vi "CreatePrivateEvents.vi"(8 "error in (no error)":errorcluster, 11 "LockinDAQ":refnum<class "Lockin.DAQ.lvclass">=refnum) -> (0 "error out":errorcluster, 3 "LockinDAQ out":refnum<class "Lockin.DAQ.lvclass">)   [LabVIEW 2016, in "Lockin.DAQ.lvclass"]
doc: "---------------------------------------------------------------\nJKI State Machine Objects™\nhttp://jki.net/state-machine-objects/\nCopyright (C) 2005-2015, JKI <info@jki.net>\nALL RIGHTS RESERVEDJKI State Machine Objects (SMO) 1.0.0.4\nJKI - JKI\nCopyright (c) 2015, JKI"
uses:
  Lockin.DAQ.lvclass
  Typedefs/PrivateEvents--Lockin.DAQ.setAOconfig.ctl
  Typedefs/AO.config-array.ctl
  Typedefs/AO.config-cluster.ctl
  Typedefs/446xAO-enum.ctl
  Typedefs/DAQType-enum.ctl
  Typedefs/PrivateEvents--Lockin.DAQ.setAIconfig.ctl
  Typedefs/AI.config-array.ctl
  Typedefs/AI.config-cluster.ctl
  Typedefs/AI.coupling-enum.ctl
  Typedefs/446xAI-enum.ctl
  Typedefs/AI Simulation-enum.ctl
  Typedefs/PrivateEvents--Lockin.DAQ.setAO.ctl
  Typedefs/AO-cluster.ctl
  Typedefs/Function-enum.ctl
  Typedefs/PrivateEvents--Lockin.DAQ.setREF.ctl
  Typedefs/REF-cluster.ctl
  Typedefs/PrivateEvents--Lockin.DAQ.setSampling.ctl
  Typedefs/Sampling.ctl
  Typedefs/Sample Mode--Ring.ctl
  Typedefs/PrivateEvents--Lockin.DAQ.setState.ctl
  Typedefs/Set State-enum.ctl
  Typedefs/PrivateEvents--Lockin.DAQ.setGain.ctl
  Typedefs/PrivateEvents--Lockin.DAQ.setSweep.ctl
  Typedefs/Sweep Configuration--Cluster.ctl
  Typedefs/Sweep Pattern--Enum.ctl
  Typedefs/PrivateEvents--Lockin.DAQ.measureOffset.ctl
  Typedefs/PrivateEvents--Lockin.DAQ.zeroOffset.ctl
  Typedefs/PrivateEvents--Lockin.DAQ.setPreFilter.ctl
  Typedefs/AI Prefilter-cluster.ctl
  Typedefs/PrivateEvents--Lockin.DAQ.autoContigureDAQ.ctl
  Typedefs/PrivateEvents--LockinDAQ.setCalibration.ctl
  Lockin.DAQ.lvclass/Lockin.DAQ.ctl
  Typedefs/PrivateEvents--LockinDAQ.Calibrate.ctl
  <vilib>/JKI/JKI SMO/SMO/SMO.lvclass
panel:
  # "For instructions on how to use the JKI State Machine Objects, examples and video tutorials, visit:\nhttp://jki.net/state-machine-objects/\n\nJKI State Machine Objects™\nhttp://jki.net/state-machine-objects/\nCopyright (C) 2005-2015, JKI <info@jki.net>\nALL RIGHTS RESERVED"
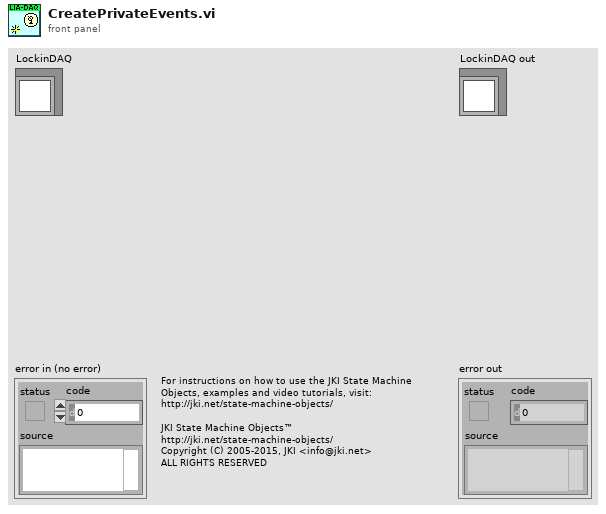
[diagram p1: front panel]
types:
  T1 = typedef "Lockin.DAQ.lvclass/PrivateEvents--LockinDAQ.setCalibration.ctl" = bool
  T2 = typedef "PrivateEvents--LockinDAQ.Calibrate.ctl" = bool
  T3 = typedef "Lockin.DAQ.lvclass/PrivateEvents--Lockin.DAQ.autoContigureDAQ.ctl" = bool
  T4 = typedef "Lockin.DAQ.lvclass/PrivateEvents--Lockin.DAQ.setPreFilter.ctl" = cluster{"PreFilter":T5}
  T5 = typedef "Lockin.DAQ.lvclass/AI Prefilter-cluster.ctl" = cluster{"60 Hz prefilter":bool, "LP prefilter":bool, "LP cutoff (Hz)":dbl}
  T6 = typedef "Lockin.DAQ.lvclass/PrivateEvents--Lockin.DAQ.zeroOffset.ctl" = bool
  T7 = typedef "Lockin.DAQ.lvclass/PrivateEvents--Lockin.DAQ.measureOffset.ctl" = bool
  T8 = typedef "Lockin.DAQ.lvclass/PrivateEvents--Lockin.DAQ.setSweep.ctl" = cluster{"setSweep":T9}
  T9 = typedef "Lockin.DAQ.lvclass/Sweep Configuration--Cluster.ctl" = cluster{"Sweep Lockin Time (s)":dbl, "Sweep IV Step (V)":dbl, "Initial Wait Time (s)":dbl, "Sweep Channel":i32[], "Sweep Start (V)":dbl[], "Sweep End (V)":dbl[], "Pattern":T10[], "Return to Start":bool}
  T10 = typedef "Lockin.DAQ.lvclass/Sweep Pattern--Enum.ctl" = enum16{"Ramp", "Ramp (RTS)", "Smooth Ramp", "Smooth Ramp (RTS)", "Frequency"}
  T11 = typedef "Lockin.DAQ.lvclass/PrivateEvents--Lockin.DAQ.setGain.ctl" = dbl[]
  T12 = typedef "Lockin.DAQ.lvclass/PrivateEvents--Lockin.DAQ.setState.ctl" = cluster{"setState":T13}
  T13 = typedef "Lockin.DAQ.lvclass/Set State-enum.ctl" = enum16{"start", "stop", "reset", "start sweep", "stop sweep"}
  T14 = typedef "Lockin.DAQ.lvclass/PrivateEvents--Lockin.DAQ.setSampling.ctl" = cluster{"Sampling":T15, "Sample Mode":T16, "AI Buffer Size (S)":i32, "Decimation":i32}
  T15 = typedef "Lockin.DAQ.lvclass/Sampling.ctl" = cluster{"Fs":dbl, "#s":i32}
  T16 = typedef "Lockin.DAQ.lvclass/Sample Mode--Ring.ctl" = i32
  T17 = typedef "Lockin.DAQ.lvclass/PrivateEvents--Lockin.DAQ.setREF.ctl" = cluster{"Channels: Lockin":T18}
  T18 = typedef "Lockin.DAQ.lvclass/REF-cluster.ctl" = cluster{"Ch":i32[], " f (Hz)":dbl[], "Phase (°)":dbl[], "TC (s)":dbl[], "order":i32[]}
  T19 = typedef "Lockin.DAQ.lvclass/PrivateEvents--Lockin.DAQ.setAO.ctl" = cluster{"Channels: AO":T20}
  T20 = typedef "Lockin.DAQ.lvclass/AO-cluster.ctl" = cluster{"Ch":i32[], "Amp (V)":dbl[], "DC (V)":dbl[], "f (Hz)":dbl[], "Phase (°)":dbl[], "Function":T21[], "Sweep?":bool[]}
  T21 = typedef "Lockin.DAQ.lvclass/Function-enum.ctl" = enum16{"Sine", "Triangle", "Square", "Sawtooth"}
  T22 = typedef "Lockin.DAQ.lvclass/PrivateEvents--Lockin.DAQ.setAIconfig.ctl" = cluster{"AI Configuration":T23, "Simulation mode":T28}
  T23 = typedef "Lockin.DAQ.lvclass/AI.config-array.ctl" = T24[]
  T24 = typedef "Lockin.DAQ.lvclass/AI.config-cluster.ctl" = cluster{"AI.channels":tag, "AI.Coupling":T25, "AI.Range":T26, "input terminal configuration":i32, "DAQ Type":T27}
  T25 = typedef "Lockin.DAQ.lvclass/AI.coupling-enum.ctl" = u16
  T26 = typedef "Lockin.DAQ.lvclass/446xAI-enum.ctl" = enum16{"±0.316 V", "±1.00 V", "±3.16 V", "±10.0 V", "±31.6 V", "±42.4 V"}
  T27 = typedef "Lockin.DAQ.lvclass/DAQType-enum.ctl" = enum16{"None", "USB 4431", "PXI 446x"}
  T28 = typedef "Lockin.DAQ.lvclass/AI Simulation-enum.ctl" = enum16{"AI = HW simulated", "AI = noise*AO", "AI = waveguide"}
  T29 = typedef "Lockin.DAQ.lvclass/PrivateEvents--Lockin.DAQ.setAOconfig.ctl" = cluster{"AO Configuration":T30}
  T30 = typedef "Lockin.DAQ.lvclass/AO.config-array.ctl" = T31[]
  T31 = typedef "Lockin.DAQ.lvclass/AO.config-cluster.ctl" = cluster{"AO.channels":tag, "AO.Range":T32, "output terminal configuration":i32, "DAQ Type":T27}
  T32 = typedef "Lockin.DAQ.lvclass/446xAO-enum.ctl" = enum16{"±0.1 V", "±1.0 V", "±10.0 V"}
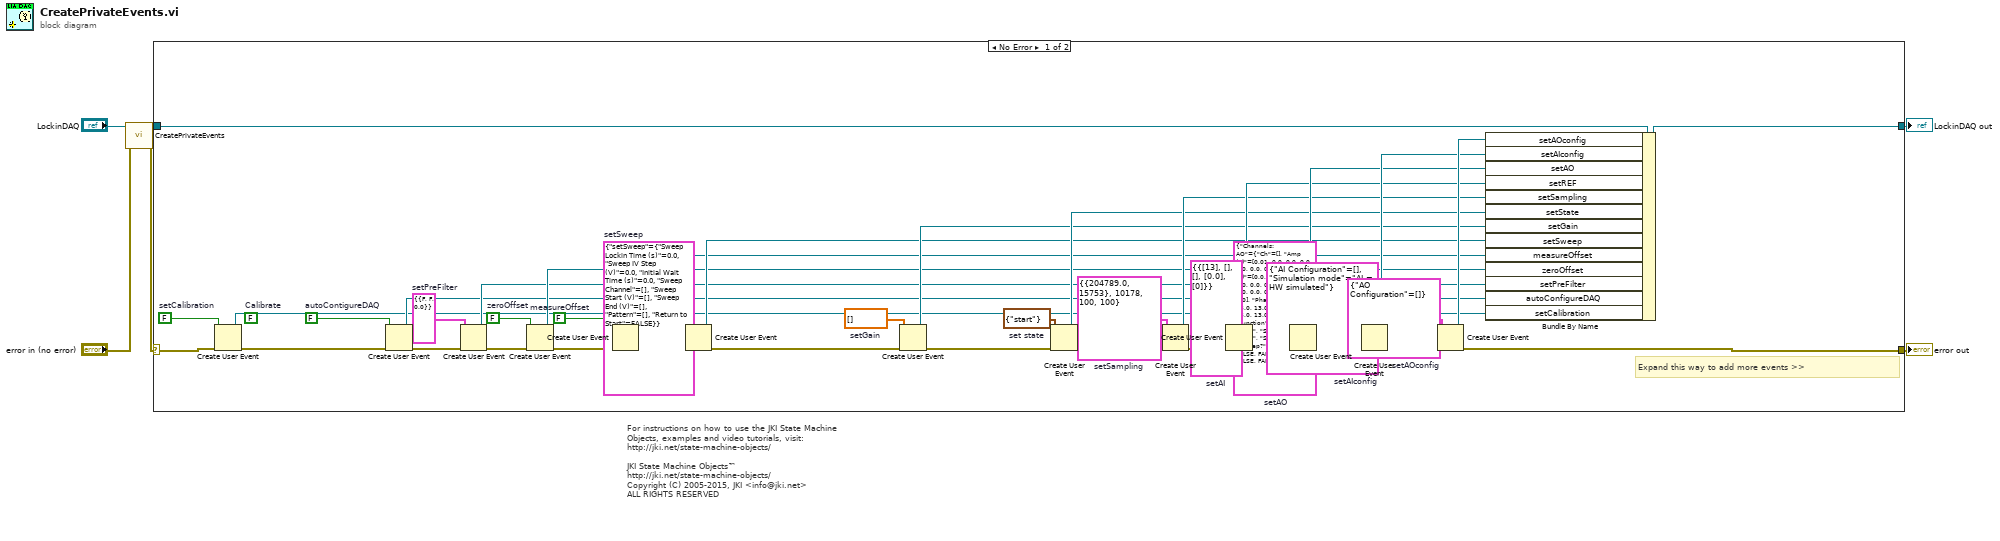
[diagram p0: block diagram]
diagram:
  # "For instructions on how to use the JKI State Machine Objects, examples and video tutorials, visit:\nhttp://jki.net/state-machine-objects/\n\nJKI State Machine Objects™\nhttp://jki.net/state-machine-objects/\nCopyright (C) 2005-2015, JKI <info@jki.net>\nALL RIGHTS RESERVED"
  n1 = call-parent "CreatePrivateEvents.vi"("error in (no error)"="error in (no error)", "SMO"="LockinDAQ") -> ("error out"=w1:errorcluster, "SMO out"=w3:refnum<class "Lockin.DAQ.lvclass">)  [unwired: 8 in]
  n2 = case shown="No Error" w1 {
    selector: w1 -> [w10 w50]
    tunnel: [w46 w50] -> w5
    tunnel: [w47 w49] -> w6
    tunnel: w3 -> [w48 w49]
    frame No Error {
      w8 = T1 FALSE  # setCalibration
      (unwired) T2 FALSE  # Calibrate
      w12 = T3 FALSE  # autoContigureDAQ
      w15 = T4 {"PreFilter"={"60 Hz prefilter"=FALSE, "LP prefilter"=FALSE, "LP cutoff (Hz)"=0.0}}  # setPreFilter
      w18 = T6 FALSE  # zeroOffset
      w21 = T7 FALSE  # measureOffset
      w24 = T8 {"setSweep"={"Sweep Lockin Time (s)"=0.0, "Sweep IV Step (V)"=0.0, "Initial Wait Time (s)"=0.0, "Sweep Channel"=[], "Sweep Start (V)"=[], "Sweep End (V)"=[], "Pattern"=[], "Return to Start"=FALSE}}  # setSweep
      w27 = T11 []  # setGain
      w30 = T12 {"setState"=enum."start"}  # set state
      w33 = T14 {"Sampling"={"Fs"=204789.0, "#s"=15753}, "Sample Mode"=10178, "AI Buffer Size (S)"=100, "Decimation"=100}  # setSampling
      w36 = T17 {"Channels: Lockin"={"Ch"=[13], " f (Hz)"=[], "Phase (°)"=[], "TC (s)"=[0.0], "order"=[0]}}  # setAI
      w39 = T19 {"Channels: AO"={"Ch"=[], "Amp (V)"=[0.01, 0.0, 0.0, 0.0, 0.0, 0.0, 0.0, 0.0], "DC (V)"=[0.0, 0.0, 0.0, 0.0, 0.0, 0.0, 0.0, 0.0], "f (Hz)"=[0.0, 0.0, 0.0, 0.0, 0.0, 0.0, 0.0, 0.0], "Phase (°)"=[13.1, 13.0, 13.0, 13.0, 13.0, 13.0, 13.0, 13.0], "Function"=[enum."Sine", enum."Sine", enum."Sine", enum."Sine", enum."Sine", enum."Sine", enum."Sine", enum."Sine"], "Sweep?"=[FALSE, FALSE, FALSE, FALSE, FALSE, FALSE, FALSE, FALSE]}}  # setAO
      w42 = T22 {"AI Configuration"=[], "Simulation mode"=enum."AI = HW simulated"}  # setAIconfig
      w45 = T29 {"AO Configuration"=[]}  # setAOconfig
      # "Expand this way to add more events >>"
      n3 = Create User Event(user event datatype=w8, error in=w10) -> (user event=w7:refnum<user-event>, error out=w9:errorcluster)
      n4 = Create User Event(user event datatype=w12, error in=w9) -> (user event=w11:refnum<user-event>, error out=w13:errorcluster)
      n5 = Create User Event(user event datatype=w15, error in=w13) -> (user event=w14:refnum<user-event>, error out=w16:errorcluster)
      n6 = Create User Event(user event datatype=w18, error in=w16) -> (user event=w17:refnum<user-event>, error out=w19:errorcluster)
      n7 = Create User Event(user event datatype=w21, error in=w19) -> (user event=w20:refnum<user-event>, error out=w22:errorcluster)
      n8 = Create User Event(user event datatype=w24, error in=w22) -> (user event=w23:refnum<user-event>, error out=w25:errorcluster)
      n9 = Create User Event(user event datatype=w27, error in=w25) -> (user event=w26:refnum<user-event>, error out=w28:errorcluster)
      n10 = Create User Event(user event datatype=w30, error in=w28) -> (user event=w29:refnum<user-event>, error out=w31:errorcluster)
      n11 = Create User Event(user event datatype=w33, error in=w31) -> (user event=w32:refnum<user-event>, error out=w34:errorcluster)
      n12 = Create User Event(user event datatype=w36, error in=w34) -> (user event=w35:refnum<user-event>, error out=w37:errorcluster)
      n13 = Create User Event(user event datatype=w39, error in=w37) -> (user event=w38:refnum<user-event>, error out=w40:errorcluster)
      n14 = Create User Event(user event datatype=w42, error in=w40) -> (user event=w41:refnum<user-event>, error out=w43:errorcluster)
      n15 = Create User Event(user event datatype=w45, error in=w43) -> (user event=w44:refnum<user-event>, error out=w46:errorcluster)
      n16 = Bundle By Name(cluster=w48, "setAOconfig"=w44, "setAIconfig"=w41, "setAO"=w38, "setREF"=w35, "setSampling"=w32, "setState"=w29, "setGain"=w26, "setSweep"=w23, "measureOffset"=w20, "zeroOffset"=w17, "setPreFilter"=w14, "autoConfigureDAQ"=w11, "setCalibration"=w7) -> (w47:refnum<class "Lockin.DAQ.lvclass">)
    }
    frame Error {
    }
  }
  "error out" <- w5
  "LockinDAQ out" <- w6
